vi "Lab.05_DAQ_1-2.vi"() -> ()   [LabVIEW 2016]
uses:
  <vilib>/Analysis/NI_AAL_SigProc.lvlib
panel:
  out "input signal":dynamicdata(graph)
  out "calculated running time":dbl
  out "frequency in a loop":dbl
  out "frequency in running time":dbl
  out "# of peak in running time":dbl
  out "# of peak in a loop":dbl
  out "running time":dbl
  out "iteration":i32
  in  "stop":bool
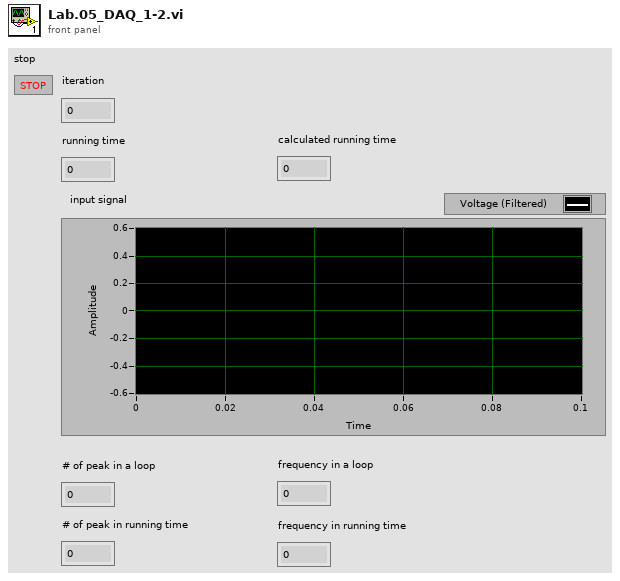
[diagram p1: front panel]
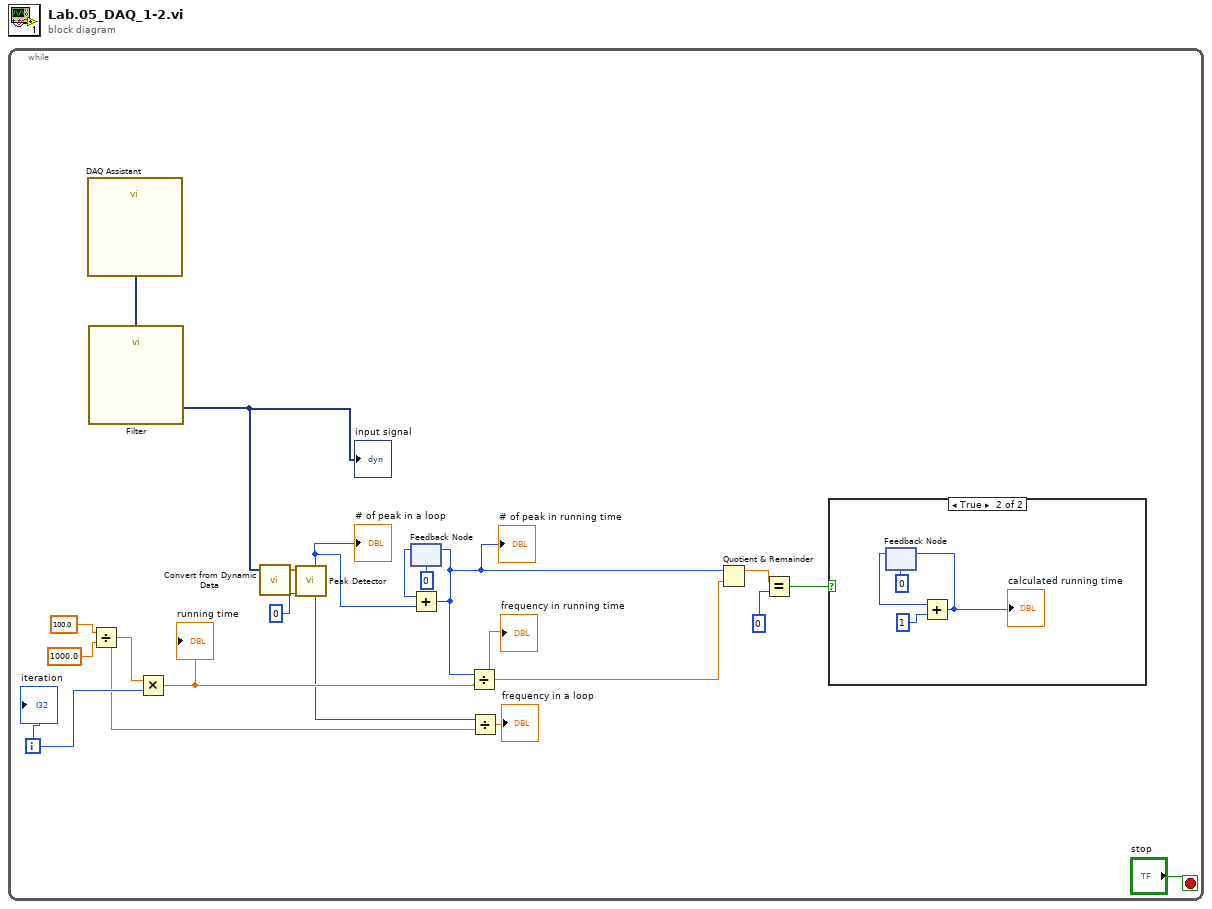
[diagram p0: block diagram]
diagram:
  n1 = while {
    i -> [w10]
    stop <- "stop" stop-if-true
    n2 = call "DAQ Assistant"() -> ("data"=w16:dynamicdata)  [unwired: 17 in, 2 out]
    n3 = call "Filter"("Signal"=w16) -> ("Filtered Signal"=w1:dynamicdata)  [unwired: 9 in, 1 out]
    "input signal" <- w1
    n4 = Divide(x=100.0, y=1000.0) -> (x/y=w7:dbl)
    n5 = Multiply(x=w7, y=w10) -> (x*y=w11:dbl)
    "running time" <- w11
    n6 = call "Convert from Dynamic Data"("Dynamic Data Type"=w1) -> ("Array"=w15:dbl[])  [unwired: 3 in]
    n7 = call <vilib>:"Peak Detector.vi"("peaks/valleys"=0, "X"=w15) -> ("# found"=w9:i32)  [unwired: 5 in, 4 out]
    "# of peak in a loop" <- w9
    n8 = feedback #1(0) -> (w13:i32)
    n9 = Add(x=w13, y=w9) -> (x+y=w6:i32)
    "# of peak in running time" <- w6
    n10 = feedback-in #1(w6) -> ()
    n11 = Divide(x=w6, y=w11) -> (x/y=w5:dbl)
    "frequency in running time" <- w5
    n12 = Divide(x=w9, y=w7) -> (x/y=→"frequency in a loop":dbl)
    n13 = Quotient & Remainder(x=w6, y=w5) -> (x-y*floor(x/y)=w2:dbl)  [unwired: 1 out]
    n14 = Equal?(x=w2, y=0) -> (x = y?=w3:bool)
    n15 = case shown="True" w3 {
      frame False {
      }
      frame True {
        n16 = feedback #2(0) -> (w22:i32)
        n17 = Add(x=w22, y=1) -> (x+y=w20:i32)
        "calculated running time" <- w20
        n18 = feedback-in #2(w20) -> ()
      }
    }
    "iteration" <- w10
  }
